vi "Get Status Source.vi"(8 "error in (no error)":errorcluster, 11 "VISA resource name in":refnum<visa-resource-name>) -> (0 "error out":errorcluster, 2 "Status Source":T1, 3 "VISA resource name":refnum<visa-resource-name>)   [LabVIEW 2020, in "CTI-Visa.lvlib"]
uses:
  CTI-Visa.lvlib
  Status Source.ctl
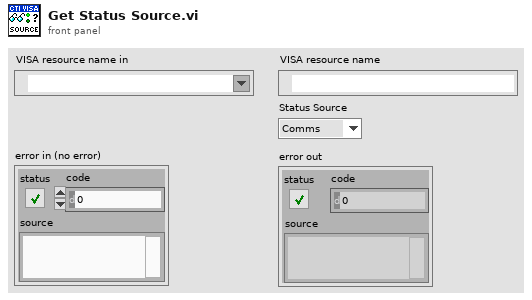
[diagram p1: front panel]
types:
  T1 = typedef "CTI-Visa.lvlib/Status Source.ctl" = enum16{"Comms", "User"}
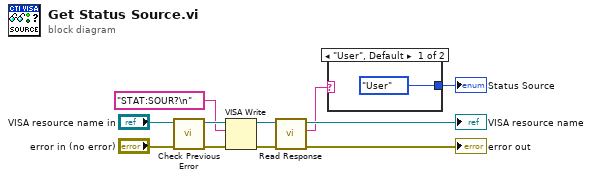
[diagram p0: block diagram]
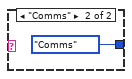
[diagram p2: hidden frame]
diagram:
  n1 = call "Check Previous Error.vi"("error in (no error)"="error in (no error)", "VISA resource name in"="VISA resource name in") -> ("error out"=w10:errorcluster, "VISA resource name"=w11:refnum<visa-resource-name>)  [unwired: 8 in]
  n2 = VISA Write(VISA resource name=w11, write buffer="STAT:SOUR?\n" ("format string"), error in (no error)=w10) -> (VISA resource name out=w8:refnum<visa-resource-name>, error out=w9:errorcluster)  [unwired: 1 out]
  n3 = call "Read Response.vi"("error in (no error)"=w9, "VISA resource name in"=w8) -> ("error out"=→"error out":errorcluster, "Response"=w3:string, "VISA resource name"=→"VISA resource name":refnum<visa-resource-name>)  [unwired: 7 in]
  n4 = case shown="\"User\", Default" w3 {
    tunnel: [Status_Source."User" ("Status Source") Status_Source."Comms" ("Status Source")] -> w1
    frame "User", Default {
    }
    frame "Comms" {
    }
  }
  "Status Source" <- w1
